vi "Create Message Data Clusters (simple).vi"(8 "error in (no error)":errorcluster, 10 "Message Metadata":T1, 11 "LVClassLibrary in":refnum<vi>) -> (0 "error out":errorcluster, 3 "LVClassLibrary out":refnum<vi>)   [LabVIEW 2019, in "gRPC Scripting Tools.lvlib"]
uses:
  gRPC Scripting Tools.lvlib
  TypeDefs/Message Metadata (Scripting).ctl
  TypeDefs/Message Element Metadata (Scripting).ctl
  TypeDefs/Message Element Type.ctl
  <vilib>/Utility/miscctls.llb/LVPositionTypeDef.ctl
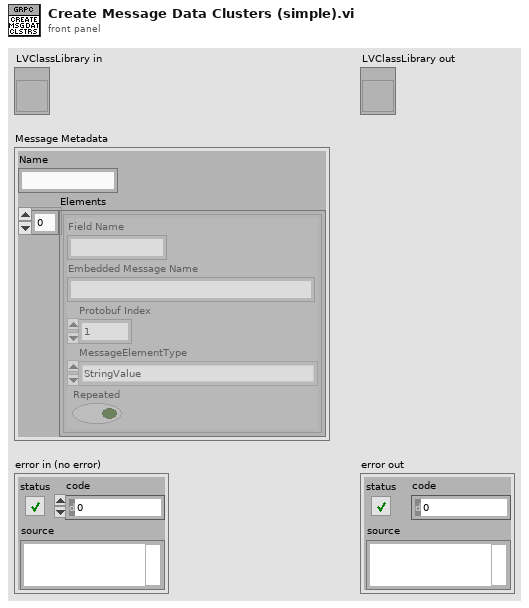
[diagram p1: front panel]
types:
  T1 = typedef "gRPC Scripting Tools.lvlib/Message Metadata (Scripting).ctl" = cluster{"Name":string, "Elements":T2[]}
  T2 = typedef "gRPC Scripting Tools.lvlib/Message Element Metadata (Scripting).ctl" = cluster{"Field Name":string, "Embedded Message Name":string, "Protobuf Index":i32, "MessageElementType":T3, "Repeated":bool}
  T3 = typedef "gRPC Scripting Tools.lvlib/Message Element Type.ctl" = enum32{"Int32Value", "FloatValue", "DoubleValue", "BoolValue", "StringValue", "MessageValue", ""}
  T4 = typedef "LVPositionTypeDef.ctl" = cluster{"Left":i32, "Top":i32}
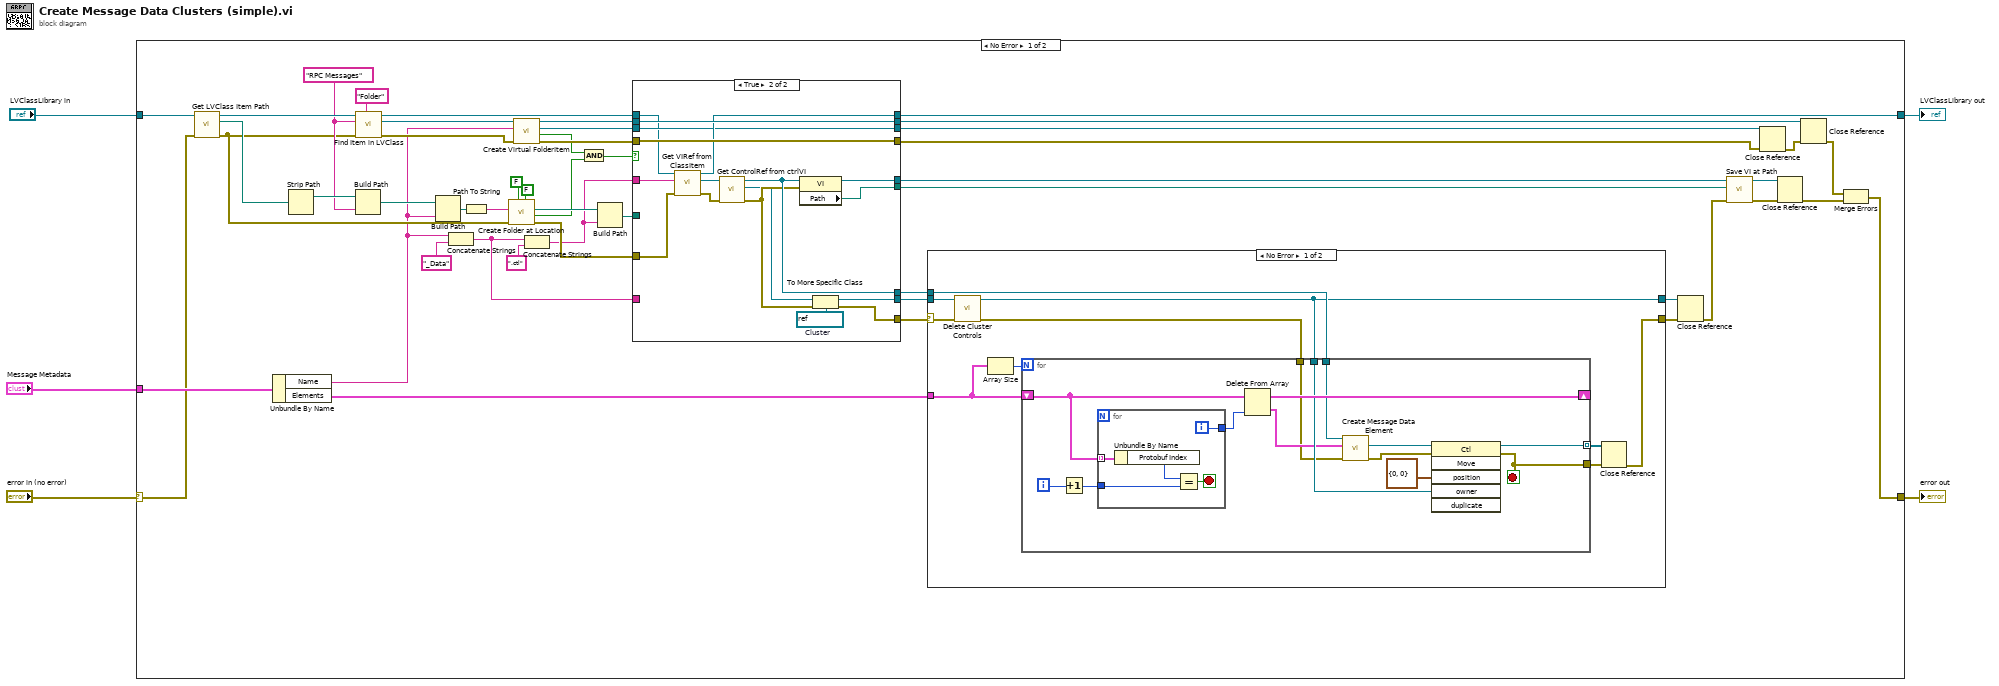
[diagram p0: block diagram]
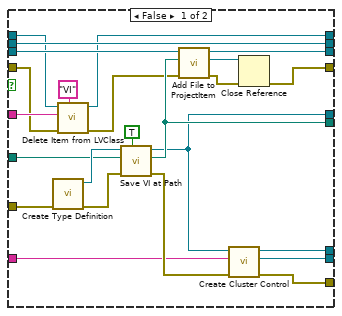
[diagram p2: hidden frame]
diagram:
  n1 = case shown="No Error" "error in (no error)" {
    selector: "error in (no error)" -> [w27 w128]
    tunnel: "Message Metadata" -> [w55 _]
    tunnel: "LVClassLibrary in" -> [w46 w129]
    tunnel: [w30 w128] -> w3
    tunnel: [w17 w129] -> w2
    frame No Error {
      w34 = "RPC Messages" ("Item Name")
      n2 = call "Get LVClass Item Path.vi"("error in (no error)"=w27, "LVClassLibrary in"=w46) -> ("error out"=w33:errorcluster, "Path"=w47:path, "LVClassLibrary out"=w35:refnum<vi>)  [unwired: 7 in]
      n3 = Unbundle By Name(w55) -> ("Name"=w23:string, "Elements"=w41:T2[])
      n4 = Strip Path(path=w47) -> (stripped path=w48:path)  [unwired: 1 out]
      n5 = Build Path(base path=w48, name or relative path=w34) -> (appended path=w50:path)
      n6 = call "Find Item in LVClass.vi"("Item Type"="Folder", "error in (no error)"=w33, "Item Name"=w34, "Class Item in"=w35) -> ("error out"=w32:errorcluster, "Project Item (Class Item)"=w36:refnum<vi>, "Class Item out"=w18:refnum<vi>)  [unwired: 4 in, 1 out]
      n7 = Build Path(base path=w50, name or relative path=w23) -> (appended path=w51:path)
      n8 = Concatenate Strings(w23, "_Data" ("string")) -> (w6:string)
      n9 = Path To String(path=w51) -> (string=w53:string)
      n10 = call "Create Folder at Location.vi"("Override existing (F)"=FALSE, "Use Relative (F)"=FALSE ("Use Relative"), "Error In"=w33, "Path"=w53) -> ("Error Out"=w52:errorcluster, "Already Exists ?"=w10:bool, "Full path out"=w54:path)  [unwired: 5 in]
      n11 = call "Create Virtual FolderItem.vi"("error in (no error)"=w32, "Folder Name"=w23, "ProjectItem in"=w36) -> ("error out"=w14:errorcluster, "Already exists?"=w11:bool, "FolderItem reference out"=w20:refnum<vi>, "ProjectItem out"=w19:refnum<vi>)  [unwired: 5 in]
      n12 = Concatenate Strings(w6, ".ctl" ("string")) -> (w7:string)
      n13 = And(x=w11, y=w10) -> (x .and. y?=w9:bool)
      n14 = Build Path(base path=w54, name or relative path=w7) -> (appended path=w21:path)
      n15 = case shown="True" w9 {
        tunnel: w52 -> [w79 w85]
        tunnel: [w64 w89] -> w44
        tunnel: [w78 w82] -> w43
        tunnel: [w77 w94] -> w42
        tunnel: [w76 w95] -> w40
        tunnel: w21 -> [w73 _]
        tunnel: w20 -> [w71 w87]
        tunnel: w19 -> [w75 w96]
        tunnel: w18 -> [w62 w86]
        tunnel: [w60 w91] -> w17
        tunnel: [w75 w96] -> w16
        tunnel: [w69 w87] -> w13
        tunnel: w7 -> [w61 w88]
        tunnel: [w70 w90] -> w15
        tunnel: w14 -> [w59 w92]
        tunnel: [w66 w92] -> w12
        tunnel: w6 -> [w56 _]
        frame False {
          n16 = call "Create Type Definition.vi"("error in (no error)"=w79) -> ("error out"=w72:errorcluster, "TypeDef VI out"=w74:refnum<vi>)  [unwired: 9 in]
          n17 = call "Delete Item from LVClass.vi"("Item Type"="VI", "error in (no error)"=w59, "Item name"=w61, "LVClassLibrary in"=w62) -> ("error out"=w58:errorcluster, "LVClassLibrary out"=w60:refnum<vi>)  [unwired: 5 in, 1 out]
          n18 = call "Save VI at Path.vi"("Override Existing? (T)"=TRUE, "error in (no error)"=w72, "Path"=w73, "VI in"=w74) -> ("error out"=w65:errorcluster, "Path to saved File"=w70:path, "VI out"=w64:refnum<vi>)  [unwired: 5 in]
          n19 = call "Add File to ProjectItem.vi"("error in (no error)"=w58, "File Path"=w70, "ProjectItem in"=w71) -> ("error out"=w68:errorcluster, "Added File ref"=w67:refnum<vi>, "ProjectItem out"=w69:refnum<vi>)  [unwired: 6 in]
          n20 = call "Create Cluster Control.vi"("error in (no error)"=w65, "Cluster Label"=w56, "Owning vi in"=w64) -> ("error out"=w76:errorcluster, "Cluster ref out"=w77:refnum<vi>, "Owning vi out"=w78:refnum<vi>)  [unwired: 6 in]
          n21 = Close Reference(reference=w67, error in (no error)=w68) -> (error out=w66:errorcluster)
        }
        frame True {
          w93 = refnum<vi> refnum  # Cluster
          n22 = call "Get VIRef from ClassItem.vi"("error in (no error)"=w85, "Item Name"=w88, "LVClassLibrary in"=w86) -> ("error out"=w83:errorcluster, "VIref out"=w84:refnum<vi>, "LVClassLibrary out"=w91:refnum<vi>)  [unwired: 5 in, 1 out]
          n23 = call "Get ControlRef from ctrlVI.vi"("error in (no error)"=w83, "VI ref in"=w84) -> ("error out"=w81:errorcluster, "Control ref out"=w80:refnum<vi>, "VI ref out"=w82:refnum<vi>)  [unwired: 7 in]
          n24 = property class="VI"(reference=w82, error in=w81) -> (reference out=w89:refnum<vi>, "Path"=w90:path)  [unwired: 1 out]
          n25 = To More Specific Class(target class=w93, reference=w80, error in=w81) -> (specific class reference=w94:refnum<vi>, error out=w95:errorcluster)
        }
      }
      n26 = case shown="No Error" w40 {
        selector: w40 -> [w99 w127]
        tunnel: [w106 w127] -> w25
        tunnel: w43 -> [w102 _]
        tunnel: w42 -> [w100 w126]
        tunnel: w41 -> [w101 _]
        tunnel: [w98 w126] -> w26
        frame No Error {
          n27 = call "Delete Cluster Controls.vi"("error in (no error)"=w99, "Cluster in"=w100) -> ("error out"=w97:errorcluster, "Cluster out"=w98:refnum<vi>)  [unwired: 8 in]
          n28 = Array Size(array=w101) -> (size(s)=w103:i32)
          n29 = for {
            N: w103 -> [_]
            shift-right: [w118] -> _
            shift-left: w101 -> [w119]
            tunnel: w98 -> [w117]
            tunnel: [w116] -> w104 mode=indexing
            tunnel: [w109] -> w105
            tunnel: w102 -> [w115]
            tunnel: w97 -> [w110]
            i -> [w108]
            stop <- w109 stop-if-true
            n30 = Increment(x=w108) -> (x+1=w107:i32)
            n31 = for {
              tunnel: w119 -> [w125] mode=indexing
              tunnel: [w123] -> w120
              tunnel: w107 -> [w121]
              i -> [w123]
              stop <- w122 stop-if-true
              n32 = Unbundle By Name(w125) -> ("Protobuf Index"=w124:i32)
              n33 = Equal?(x=w124, y=w121) -> (x = y?=w122:bool)
            }
            n34 = Delete From Array(array=w119, index=w120) -> (deleted portion=w111:T2, array with subset deleted=w118:T2[])  [unwired: 1 in]
            n35 = call "Create Message Data Element.vi"("error in (no error)"=w110, "Message Element MetaData"=w111, "Owning vi in"=w115) -> ("error out"=w112:errorcluster, "Data Element ref out (Ctrl ref)"=w113:refnum<vi>)  [unwired: 5 in, 2 out]
            n36 = invoke class="Ctl" method="Move"(reference=w113, error in=w112, "position"=T4 {"Left"=0, "Top"=0}, "owner"=w117) -> (reference out=w116:refnum<vi>, error out=w109:errorcluster)  [unwired: 2 in, 4 out]
          }
          n37 = Close Reference(reference=w104, error in (no error)=w105) -> (error out=w106:errorcluster)
        }
        frame Error {
        }
      }
      n38 = Close Reference(reference=w26, error in (no error)=w25) -> (error out=w24:errorcluster)
      n39 = call "Save VI at Path.vi"("error in (no error)"=w24, "Path"=w15, "VI in"=w44) -> ("error out"=w39:errorcluster, "VI out"=w38:refnum<vi>)  [unwired: 6 in, 1 out]
      n40 = Close Reference(reference=w13, error in (no error)=w12) -> (error out=w29:errorcluster)
      n41 = Close Reference(reference=w38, error in (no error)=w39) -> (error out=w31:errorcluster)
      n42 = Close Reference(reference=w16, error in (no error)=w29) -> (error out=w28:errorcluster)
      n43 = Merge Errors(w28, w31) -> (w30:errorcluster)
    }
    frame Error {
    }
  }
  "error out" <- w3
  "LVClassLibrary out" <- w2
